vi "多设备同步_主从.vi"() -> ()   [LabVIEW 2013]
uses:
  <userlib>/ArtDAQ/_SubVI/ArtDAQ_CreateAIVoltageChan.vi
  <userlib>/ArtDAQ/_SubVI/ArtDAQ_CfgSampClkTiming.vi
  <userlib>/ArtDAQ/_SubVI/ArtDAQ_Read Analog DBL NChan NSamp.vi
panel:
  in  "采集卡类型选择":enum16{"同步卡", "异步卡"}(ring)
  in  "从卡时钟源":string="/Dev2/PFI2"
  in  "主卡时钟导出端":string="/Dev1/PFI3"
  out "wf2":dbl[][](graph)
  out "wf":dbl[][](graph)
  in  "Stop":bool
  in  "从卡采样通道":string(combo)="Dev2/ai0"
  in  "主卡采样通道":string(combo)="Dev1/ai0"
  out "ErrorOutput":errorcluster
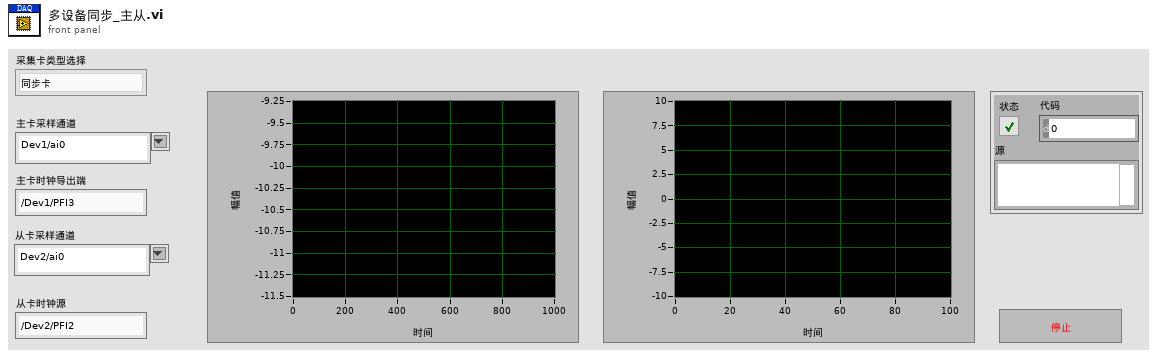
[diagram p1: front panel]
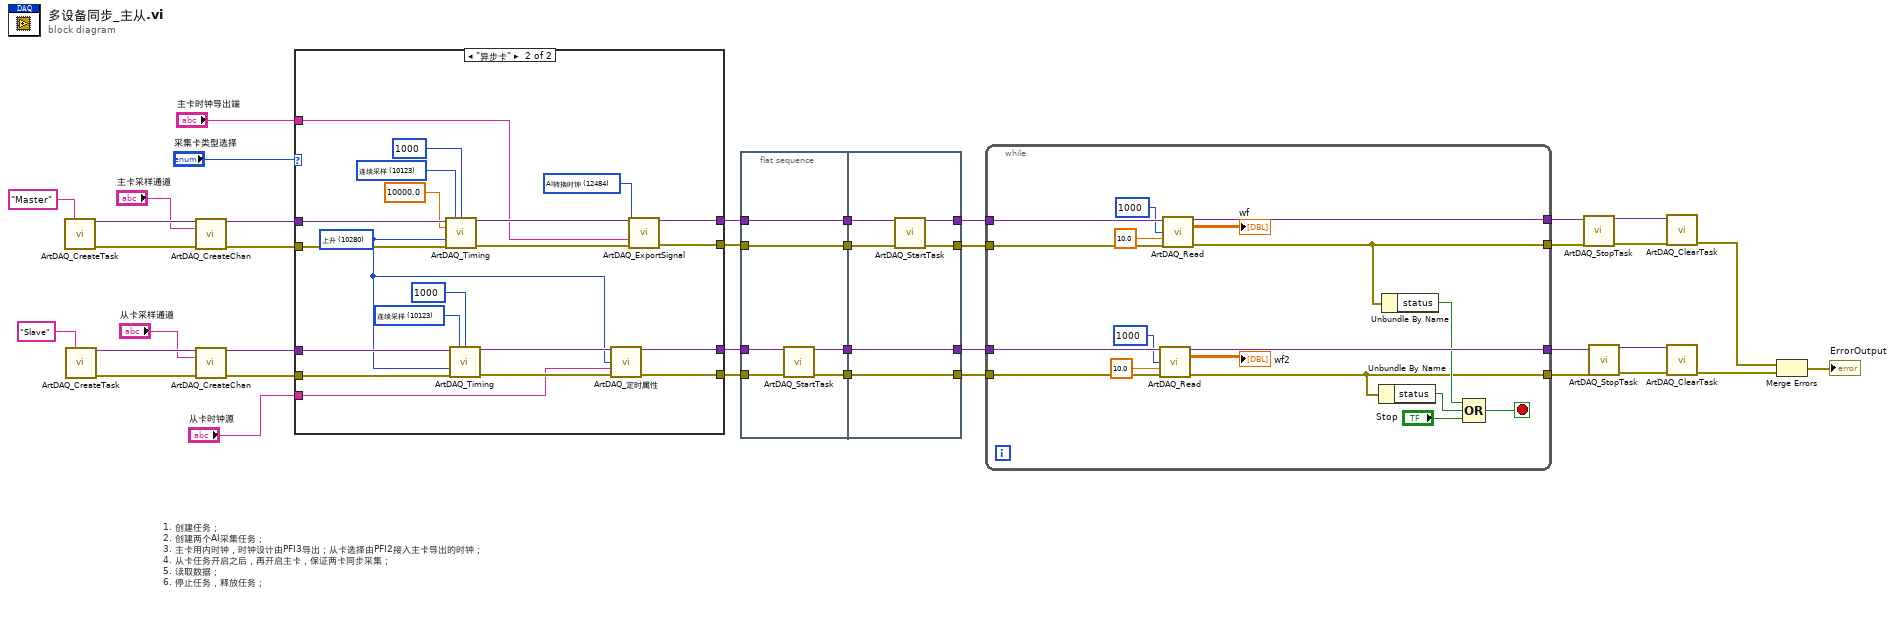
[diagram p0: block diagram]
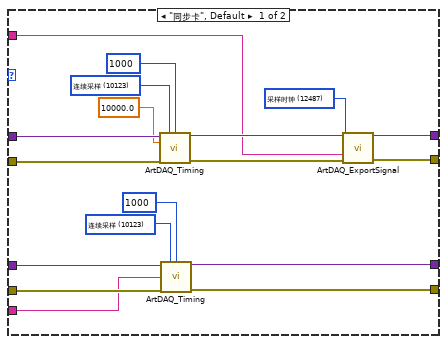
[diagram p2: hidden frame]
diagram:
  # "1. 创建任务；\n2. 创建两个AI采集任务；\n3. 主卡用内时钟，时钟设计由PFI3导出；从卡选择由PFI2接入主卡导出的时钟；\n4. 从卡任务开启之后，再开启主卡，保证两卡同步采集；\n5. 读取数据；\n6. 停止任务，释放任务；"
  n1 = call <userlib>:"ArtDAQ_CreateTask.vi"("任务名称"="Master" ("TaskName")) -> ("任务句柄"=w38:variant, "错误输出"=w37:errorcluster)  [unwired: 13 in]
  n2 = call <userlib>:"ArtDAQ_CreateTask.vi"("任务名称"="Slave" ("TaskName")) -> ("任务句柄"=w36:variant, "错误输出"=w35:errorcluster)  [unwired: 13 in]
  n3 = call-poly <userlib>:"ArtDAQ_CreateChan.vi"("任务句柄"=w38, "物理通道"="主卡采样通道", "错误输入"=w37) -> ("任务句柄"=w34:variant, "错误输出"=w33:errorcluster)  [unwired: 11 in]
  n4 = call-poly <userlib>:"ArtDAQ_CreateChan.vi"("任务句柄"=w36, "物理通道"="从卡采样通道", "错误输入"=w35) -> ("任务句柄"=w32:variant, "错误输出"=w31:errorcluster)  [unwired: 11 in]
  n5 = case shown="\"异步卡\"" "采集卡类型选择" {
    tunnel: w34 -> [w56 w77]
    tunnel: w33 -> [w55 w76]
    tunnel: w32 -> [w54 w75]
    tunnel: w31 -> [w53 w74]
    tunnel: [w48 w61] -> w7
    tunnel: [w47 w59] -> w6
    tunnel: [w44 w67] -> w5
    tunnel: [w43 w66] -> w4
    tunnel: "从卡时钟源" -> [w40 w57]
    tunnel: "主卡时钟导出端" -> [w39 w63]
    frame "同步卡", Default {
      w41 = 12487 items=["AI转换时钟"=12484, "采样时钟"=12487, "开始触发"=12491, "暂停触发"=12489, "参考触发"=12490, "计数器输出事件"=12494, "主采样时钟时基"=12495, "同步脉冲输出"=12496] ("信号")
      w42 = 10123 items=["有限点采样"=10178, "连续采样"=10123] ("采样模式")
      w51 = 10123 items=["有限点采样"=10178, "连续采样"=10123] ("采样模式")
      n6 = call-poly <userlib>:"ArtDAQ_Timing.vi"("任务句柄"=w56, "采样模式"=w51, "每通道采样数"=1000 ("SamplePerChan"), "采样率"=10000.0 ("Rate"), "错误输入"=w55) -> ("任务句柄"=w46:variant, "错误输出"=w45:errorcluster)  [unwired: 9 in]
      n7 = call-poly <userlib>:"ArtDAQ_Timing.vi"("任务句柄"=w54, "采样模式"=w42, "每通道采样数"=1000 ("SamplePerChan"), "源"=w40, "错误输入"=w53) -> ("任务句柄"=w48:variant, "错误输出"=w47:errorcluster)  [unwired: 9 in]
      n8 = call <userlib>:"ArtDAQ_ExportSignal.vi"("任务句柄"=w46, "信号"=w41, "输出接线端"=w39, "错误输入"=w45) -> ("任务句柄"=w44:variant, "错误输出"=w43:errorcluster)  [unwired: 10 in]
    }
    frame "异步卡" {
      w58 = 10280 items=["上升"=10280, "下降"=10171] ("有效边沿")
      w64 = 12484 items=["AI转换时钟"=12484, "采样时钟"=12487, "开始触发"=12491, "暂停触发"=12489, "参考触发"=12490, "计数器输出事件"=12494, "主采样时钟时基"=12495, "同步脉冲输出"=12496] ("信号")
      w65 = 10123 items=["有限点采样"=10178, "连续采样"=10123] ("采样模式")
      w72 = 10123 items=["有限点采样"=10178, "连续采样"=10123] ("采样模式")
      n9 = call-poly <userlib>:"ArtDAQ_Timing.vi"("任务句柄"=w77, "采样模式"=w72, "每通道采样数"=1000 ("SamplePerChan"), "采样率"=10000.0 ("Rate"), "有效边沿"=w58, "错误输入"=w76) -> ("任务句柄"=w69:variant, "错误输出"=w68:errorcluster)  [unwired: 8 in]
      n10 = call-poly <userlib>:"ArtDAQ_Timing.vi"("任务句柄"=w75, "采样模式"=w65, "每通道采样数"=1000 ("SamplePerChan"), "有效边沿"=w58, "错误输入"=w74) -> ("任务句柄"=w62:variant, "错误输出"=w60:errorcluster)  [unwired: 9 in]
      n11 = call-poly "ArtDAQ_定时属性.vi"("任务句柄"=w62, "边沿"=w58, "转换时钟源"=w57, "错误输入"=w60) -> ("任务句柄"=w61:variant, "错误输出"=w59:errorcluster)  [unwired: 10 in]
      n12 = call <userlib>:"ArtDAQ_ExportSignal.vi"("任务句柄"=w69, "信号"=w64, "输出接线端"=w63, "错误输入"=w68) -> ("任务句柄"=w67:variant, "错误输出"=w66:errorcluster)  [unwired: 10 in]
    }
  }
  n13 = flat-sequence {
    tunnel: w5 -> [w81]
    tunnel: w4 -> [w80]
    tunnel: w7 -> [w83]
    tunnel: w6 -> [w82]
    tunnel: [w81] -> w30
    tunnel: [w80] -> w29
    tunnel: [w79] -> w28
    tunnel: [w78] -> w27
    tunnel: w30 -> [w89]
    tunnel: w29 -> [w88]
    tunnel: w28 -> [w86]
    tunnel: w27 -> [w87]
    tunnel: [w87] -> w23
    tunnel: [w86] -> w24
    tunnel: [w85] -> w26
    tunnel: [w84] -> w25
    frame #0 {
      n14 = call <userlib>:"ArtDAQ_StartTask.vi"("任务句柄"=w83, "错误输入"=w82) -> ("任务句柄"=w79:variant, "错误输出"=w78:errorcluster)  [unwired: 12 in]
    }
    frame #1 {
      n15 = call <userlib>:"ArtDAQ_StartTask.vi"("任务句柄"=w89, "错误输入"=w88) -> ("任务句柄"=w85:variant, "错误输出"=w84:errorcluster)  [unwired: 12 in]
    }
  }
  n16 = while {
    tunnel: w26 -> [w107]
    tunnel: w25 -> [w106]
    tunnel: w24 -> [w105]
    tunnel: w23 -> [w104]
    tunnel: [w103] -> w22
    tunnel: [w98] -> w21
    tunnel: [w102] -> w20
    tunnel: [w96] -> w19
    stop <- w99 stop-if-true
    n17 = call-poly <userlib>:"ArtDAQ_Read.vi"("任务句柄"=w105, "每通道采样数"=1000 ("NumSampsPerChan"), "超时s"=10.0 ("Timeout"), "错误输入"=w104) -> ("任务句柄"=w102:variant, "数据"=→"wf2":dbl[][], "错误输出"=w96:errorcluster)  [unwired: 7 in, 2 out]
    n18 = call-poly <userlib>:"ArtDAQ_Read.vi"("任务句柄"=w107, "每通道采样数"=1000 ("NumSampsPerChan"), "超时s"=10.0 ("Timeout"), "错误输入"=w106) -> ("任务句柄"=w103:variant, "数据"=→"wf":dbl[][], "错误输出"=w98:errorcluster)  [unwired: 7 in, 2 out]
    n19 = Unbundle By Name(w96) -> ("status"=w95:bool)
    n20 = Unbundle By Name(w98) -> ("status"=w97:bool)
    n21 = Compound Arithmetic op=OR(w97, w95, "Stop") -> (w99:bool)
  }
  n22 = call <userlib>:"ArtDAQ_StopTask.vi"("任务句柄"=w22, "错误输入"=w21) -> ("任务句柄"=w18:variant, "错误输出"=w17:errorcluster)  [unwired: 12 in]
  n23 = call <userlib>:"ArtDAQ_StopTask.vi"("任务句柄"=w20, "错误输入"=w19) -> ("任务句柄"=w16:variant, "错误输出"=w15:errorcluster)  [unwired: 12 in]
  n24 = call <userlib>:"ArtDAQ_ClearTask.vi"("任务句柄"=w18, "错误输入"=w17) -> ("错误输出"=w14:errorcluster)  [unwired: 13 in]
  n25 = call <userlib>:"ArtDAQ_ClearTask.vi"("任务句柄"=w16, "错误输入"=w15) -> ("错误输出"=w13:errorcluster)  [unwired: 13 in]
  n26 = Merge Errors(w14, w13) -> (→"ErrorOutput":errorcluster)
